vi "file -- standard data file tree structure.vi"(11 "folder path":path=path "/snowfall/Users/arcadi/Desktop/Ultrasound/Experiment/YBCO_4/Round1/Sweep12/June_2011/062511/221.16400K_300_3100_001_062511.dat") -> (2 "Array":path[](array[path]))   [LabVIEW 2015]
uses:
  <vilib>/regexp/Match Regular Expression.xnode
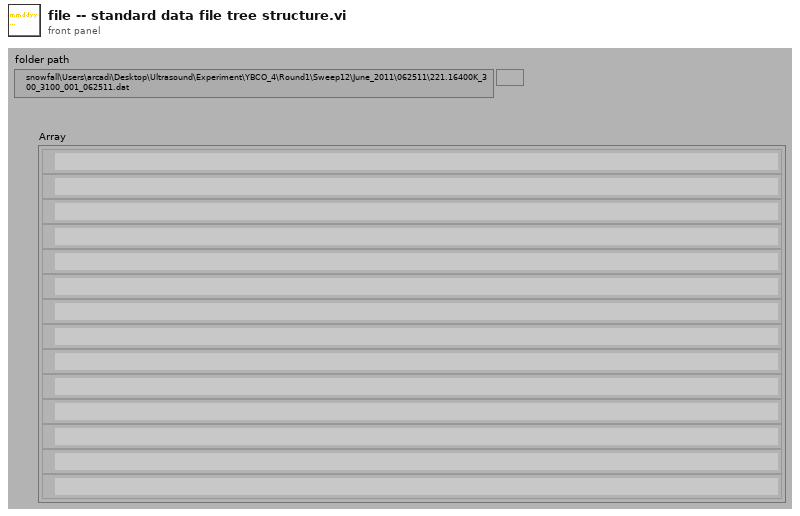
[diagram p1: front panel]
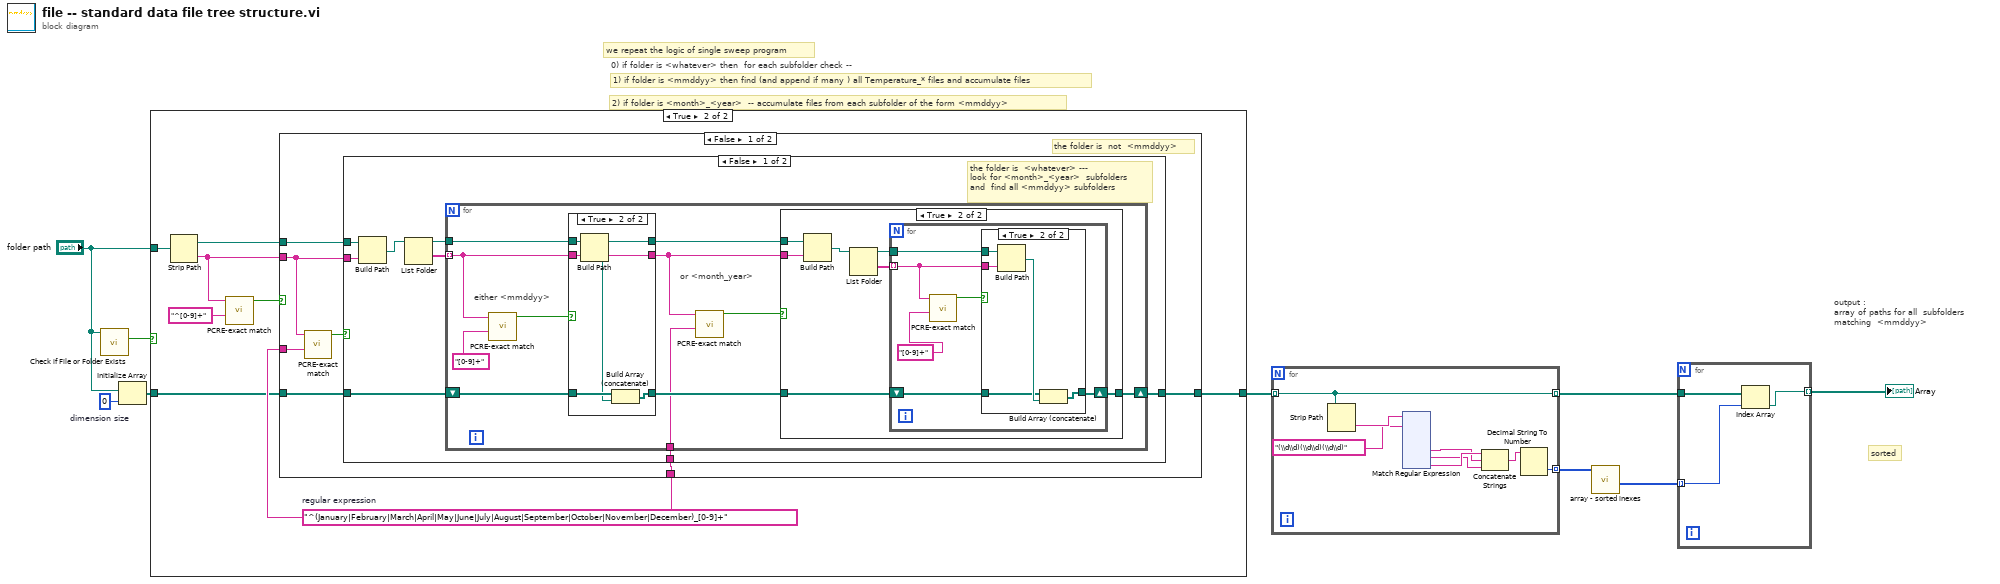
[diagram p0: block diagram]
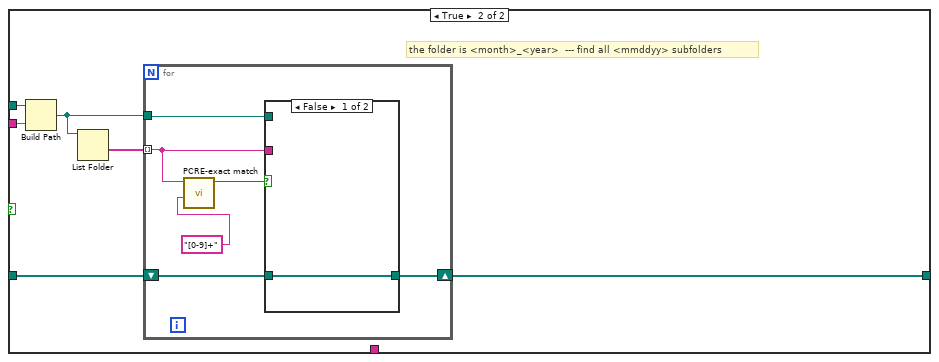
[diagram p6: hidden frame]
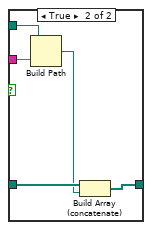
[diagram p7: hidden frame]
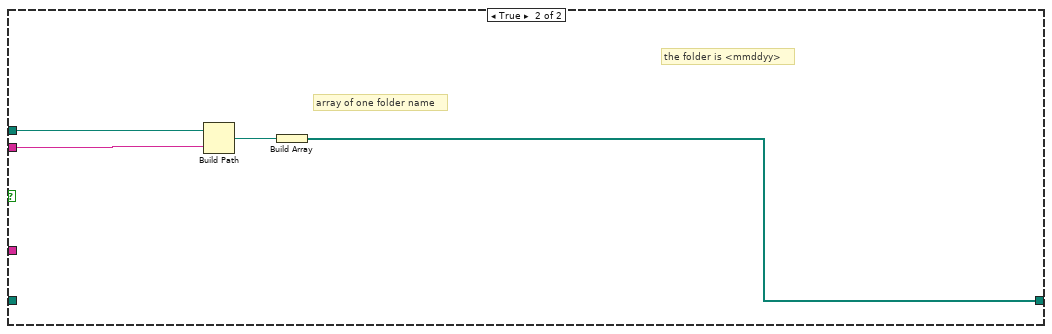
[diagram p8: hidden frame]
diagram:
  w9 = 0  # dimension size
  # "sorted"
  # "0) if folder is <whatever> then  for each subfolder check --"
  # "1) if folder is <mmddyy> then find (and append if many ) all Temperature_* files and accumulate files"
  # "2) if folder is <month>_<year>  -- accumulate files from each subfolder of the form <mmddyy>"
  # "we repeat the logic of single sweep program"
  # "output : \narray of paths for all  subfolders matching  <mmddyy>"
  n1 = call <vilib>:"Check if File or Folder Exists.vi"("path"="folder path") -> ("file or folder exists?"=w6:bool)  [unwired: 8 in, 2 out]
  n2 = Initialize Array("folder path", w9) -> (w8:path[])
  n3 = case shown="True" w6 {
    tunnel: [w10 w17] -> w5
    tunnel: w8 -> [w10 w12]
    tunnel: "folder path" -> [_ w11]
    frame False {
    }
    frame True {
      w16 = "^(January|February|March|April|May|June|July|August|September|October|November|December)_[0-9]+"  # regular expression
      n4 = Strip Path(path=w11) -> (stripped path=w18:path, name=w15:string)
      n5 = call "PCRE-exact match.vi"("regular expression"="^[0-9]+", "input string"=w15) -> ("exact match"=w13:bool)  [unwired: 7 in, 2 out]
      n6 = case shown="False" w13 {
        tunnel: [w25 w93] -> w17
        tunnel: w18 -> [w24 w92]
        tunnel: w15 -> [w20 w91]
        tunnel: w16 -> [w21 _]
        tunnel: w12 -> [w23 _]
        tunnel: w16 -> [w22 _]
        frame False {
          # "the folder is  not  <mmddyy>"
          n7 = call "PCRE-exact match.vi"("regular expression"=w21, "input string"=w20) -> ("exact match"=w19:bool)  [unwired: 7 in, 2 out]
          n8 = case shown="False" w19 {
            tunnel: [w27 w76] -> w25
            tunnel: w20 -> [w30 w75]
            tunnel: w24 -> [w31 w74]
            tunnel: w23 -> [w29 w73]
            tunnel: w22 -> [w28 _]
            frame False {
              # "the folder is  <whatever> --- \nlook for <month>_<year>  subfolders \nand  find all <mmddyy> subfolders"
              n9 = Build Path(base path=w31, name or relative path=w30) -> (appended path=w32:path)
              n10 = List Folder(path=w32) -> (path out=w26:path, folder names=w33:string[])  [unwired: 3 in, 2 out]
              n11 = for {
                tunnel: w33 -> [w39] mode=indexing
                shift-right: [w43] -> w27
                shift-left: w29 -> [w44]
                tunnel: w26 -> [w41]
                tunnel: w28 -> [w35]
                # "or <month_year>"
                # "either <mmddyy>"
                n12 = call "PCRE-exact match.vi"("regular expression"="[0-9]+", "input string"=w39) -> ("exact match"=w37:bool)  [unwired: 7 in, 2 out]
                n13 = case shown="True" w37 {
                  tunnel: w41 -> [w65 w68]
                  tunnel: w39 -> [w66 w69]
                  tunnel: w44 -> [w67 w72]
                  tunnel: [w67 w70] -> w42
                  tunnel: [w66 w69] -> w36
                  tunnel: [w65 w68] -> w40
                  frame False {
                  }
                  frame True {
                    n14 = Build Path(base path=w68, name or relative path=w69) -> (appended path=w71:path)
                    n15 = Build Array (concatenate)(w72, w71) -> (w70:path[])
                  }
                }
                n16 = call "PCRE-exact match.vi"("regular expression"=w35, "input string"=w36) -> ("exact match"=w34:bool)  [unwired: 7 in, 2 out]
                n17 = case shown="True" w34 {
                  tunnel: [w45 w48] -> w43
                  tunnel: w42 -> [w45 w49]
                  tunnel: w40 -> [_ w52]
                  tunnel: w36 -> [_ w51]
                  frame False {
                  }
                  frame True {
                    n18 = Build Path(base path=w52, name or relative path=w51) -> (appended path=w47:path)
                    n19 = List Folder(path=w47) -> (path out=w46:path, folder names=w50:string[])  [unwired: 3 in, 2 out]
                    n20 = for {
                      tunnel: w50 -> [w55] mode=indexing
                      shift-right: [w57] -> w48
                      shift-left: w49 -> [w58]
                      tunnel: w46 -> [w56]
                      n21 = call "PCRE-exact match.vi"("regular expression"="[0-9]+", "input string"=w55) -> ("exact match"=w53:bool)  [unwired: 7 in, 2 out]
                      n22 = case shown="True" w53 {
                        tunnel: w58 -> [w59 w63]
                        tunnel: [w59 w62] -> w57
                        tunnel: w56 -> [_ w61]
                        tunnel: w55 -> [_ w60]
                        frame False {
                        }
                        frame True {
                          n23 = Build Path(base path=w61, name or relative path=w60) -> (appended path=w64:path)
                          n24 = Build Array (concatenate)(w63, w64) -> (w62:path[])
                        }
                      }
                    }
                  }
                }
              }
            }
            frame True {
              # "the folder is <month>_<year>  --- find all <mmddyy> subfolders"
              n25 = Build Path(base path=w74, name or relative path=w75) -> (appended path=w77:path)
              n26 = List Folder(path=w77) -> (folder names=w78:string[])  [unwired: 3 in, 3 out]
              n27 = for {
                tunnel: w78 -> [w81] mode=indexing
                shift-right: [w82] -> w76
                shift-left: w73 -> [w83]
                tunnel: w77 -> [w84]
                n28 = call "PCRE-exact match.vi"("regular expression"="[0-9]+", "input string"=w81) -> ("exact match"=w79:bool)  [unwired: 7 in, 2 out]
                n29 = case shown="False" w79 {
                  tunnel: w84 -> [_ w90]
                  tunnel: w81 -> [_ w89]
                  tunnel: w83 -> [w85 w88]
                  tunnel: [w85 w86] -> w82
                  frame False {
                  }
                  frame True {
                    n30 = Build Path(base path=w90, name or relative path=w89) -> (appended path=w87:path)
                    n31 = Build Array (concatenate)(w88, w87) -> (w86:path[])
                  }
                }
              }
            }
          }
        }
        frame True {
          # "the folder is <mmddyy>"
          # "array of one folder name"
          n32 = Build Path(base path=w92, name or relative path=w91) -> (appended path=w94:path)
          n33 = Build Array(w94) -> (w93:path[])
        }
      }
    }
  }
  n34 = for {
    tunnel: w5 -> [w95] mode=indexing
    tunnel: [w96] -> w4 mode=indexing
    tunnel: [w95] -> w3 mode=indexing
    n35 = Strip Path(path=w95) -> (name=w102:string)  [unwired: 1 out]
    n36 = xnode "Match Regular Expression"("input string"=w102, "regular expression"="(\\d\\d)(\\d\\d)(\\d\\d)") -> ("submatch 1"=w99:string, "submatch 2"=w98:string, "submatch 3"=w100:string)  [unwired: 4 in, 5 out]
    n37 = Concatenate Strings(w100, w99, w98) -> (w97:string)
    n38 = Decimal String To Number(string=w97) -> (number=w96:i32)  [unwired: 2 in, 1 out]
  }
  n39 = call "array - sorted inexes.vi"("x"=w4) -> ("index array"=w2:i32[])  [unwired: 9 in, 1 out]
  n40 = for {
    tunnel: w3 -> [w220]
    tunnel: w2 -> [w218] mode=indexing
    tunnel: [w219] -> w1 mode=indexing
    n41 = Index Array(array=w220, index=w218) -> (element=w219:path)
  }
  "Array" <- w1
